vi "create context.vi"(8 "error in":errorcluster, 11 "thread count":u64) -> (0 "error out":errorcluster, 3 "engine context out":refnum<class "engine context.lvclass">)   [LabVIEW 2016, in "engine context.lvclass"]
uses:
  engine context.lvclass
  engine context.lvclass/engine context.ctl
  dllwrapper/library path.vi
  dllwrapper/async tls dl.lvlib
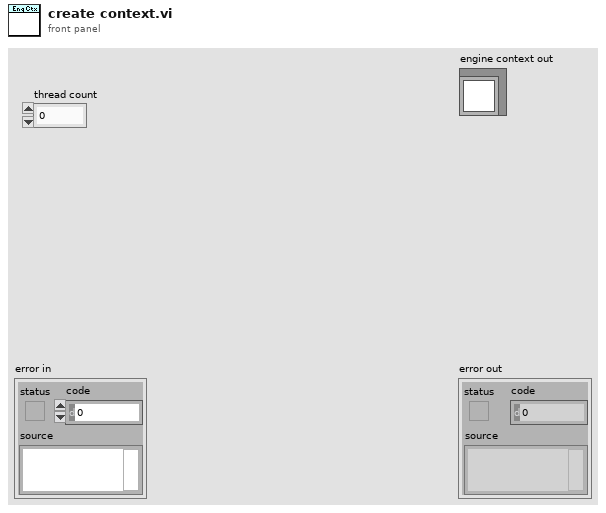
[diagram p1: front panel]
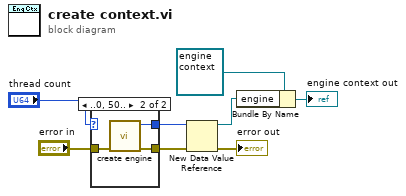
[diagram p0: block diagram]
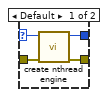
[diagram p2: hidden frame]
diagram:
  n1 = case shown="..0, 50.." "thread count" {
    selector: "thread count" -> [w9 _]
    tunnel: "error in" -> [w10 w15]
    tunnel: [w12 w14] -> w5
    tunnel: [w11 w13] -> w3
    frame Default {
      n2 = call "create nthread engine.vi"("error in"=w10, "threadCount"=w9) -> ("error out"=w12:errorcluster, "engine"=w11:u64)  [unwired: 8 in]
    }
    frame ..0, 50.. {
      n3 = call "create engine.vi"("error in"=w15) -> ("error out"=w14:errorcluster, "engine"=w13:u64)  [unwired: 9 in]
    }
  }
  n4 = New Data Value Reference(data value=w3, error in=w5) -> (data value reference=w2:refnum<data-value>, error out=→"error out":errorcluster)
  n5 = Bundle By Name(cluster=refnum<class "engine context.lvclass"> refnum ("engine context in"), "engine"=w2) -> (→"engine context out":refnum<class "engine context.lvclass">)
